vi "PH_Synchrolock_Watch.show Result.vi"(0 "i ref in":refnum<vi>, 1 "RF Current Value":dbl, 2 "Mira Current Value":dbl, 3 "Mean Phase Current Value":dbl, 5 "error in":errorcluster) -> (14 "i ref out":refnum<vi>, 19 "error out":errorcluster)   [LabVIEW 2014, in "PH_Synchrolock_Watch.lvlib"]
doc: "This VI shows the result and stores it at own attributes."
uses:
  PH_Synchrolock_Watch.lvlib
  PH_Basics/PH_Common/PH_Common.lvlib
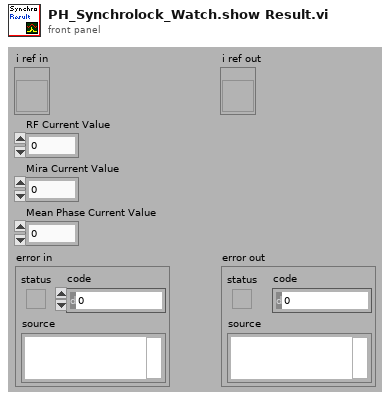
[diagram p1: front panel]
types:
  T1 = typedef "PH_Synchrolock_Watch.lvlib/PH_Synchrolock_Watch.i attribute.ctl" = cluster{"GUI Refs":cluster{"Mean Phase Graph":refnum<vi>, "RF Amplitude Graph":refnum<vi>, "Mira Amplitude Graph":refnum<vi>, "MIRA State":refnum<vi>, "Mean Phase":refnum<vi>, "RF Amplitude":refnum<vi>, "Mira Amplitude":refnum<vi>, "Mean Phase in range?":refnum<vi>, "RF Amplitude above limit?":refnum<vi>, "Mira Amplitude in range?":refnum<vi>, "Mean phase upper limit":refnum<vi>, "Mean phase lower limit":refnum<vi>, "RF Amplitude lower limit":refnum<vi>, "Mira Amplitude lower limit":refnum<vi>, "Mira Amplitude upper limit":refnum<vi>, "Mira scope":refnum<vi>, "Reset Mira warning":refnum<vi>}, "Status":cluster{"Reset Warning":bool}, "Mean Phase":cluster{"Current Value":dbl, "Upper Limit":dbl, "Lower Limit":dbl, "Data":cluster{dbl[], dbl[]}}, "RF":cluster{"Current Value":dbl, "Lower Limit":dbl, "Data":cluster{dbl[], dbl[]}}, "MIRA":cluster{"Current Value":dbl, "Upper Limit":dbl, "Lower Limit":dbl, "Data":cluster{dbl[], dbl[]}}}
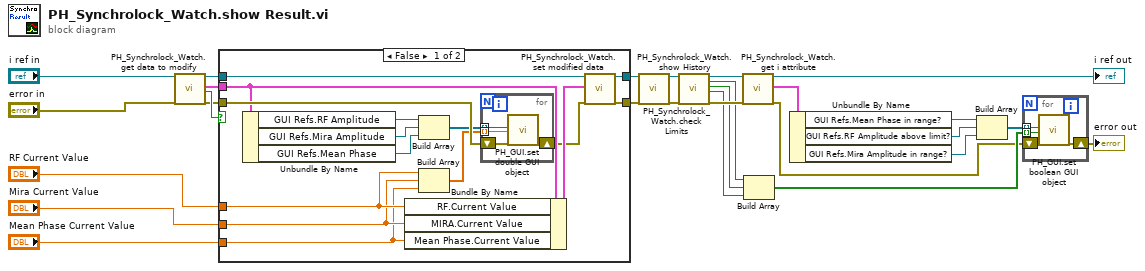
[diagram p0: block diagram]
diagram:
  n1 = call "PH_Synchrolock_Watch.get data to modify.vi"("i ref in"="i ref in", "error in (no error)"="error in") -> ("i ref out"=w23:refnum<vi>, "i attribute"=w27:T1, "timed out"=w26:bool, "error out"=w24:errorcluster)  [unwired: 14 in]
  n2 = case shown="False" w26 {
    tunnel: w23 -> [w42 w48]
    tunnel: [w41 w48] -> w3
    tunnel: w24 -> [w40 w47]
    tunnel: [w39 w47] -> w1
    tunnel: w27 -> [w37 _]
    tunnel: "RF Current Value" -> [w31 _]
    tunnel: "Mira Current Value" -> [w30 _]
    tunnel: "Mean Phase Current Value" -> [w29 _]
    frame False {
      n3 = Unbundle By Name(w37) -> ("GUI Refs.RF Amplitude"=w36:refnum<vi>, "GUI Refs.Mira Amplitude"=w35:refnum<vi>, "GUI Refs.Mean Phase"=w34:refnum<vi>)
      n4 = Bundle By Name(cluster=w37, "RF.Current Value"=w31, "MIRA.Current Value"=w30, "Mean Phase.Current Value"=w29) -> (w38:T1)
      n5 = Build Array(w36, w35, w34) -> (w33:refnum<vi>[])
      n6 = Build Array(w31, w30, w29) -> (w28:dbl[])
      n7 = for {
        shift-right: [w43] -> w32
        shift-left: w40 -> [w46]
        tunnel: w33 -> [w45] mode=indexing
        tunnel: w28 -> [w44] mode=indexing
        n8 = call "PH_GUI.set double GUI object.vi"("GUI object Ref"=w45, "value"=w44, "error in (no error)"=w46) -> ("error out"=w43:errorcluster)  [unwired: 16 in]
      }
      n9 = call "PH_Synchrolock_Watch.set modified data.vi"("i ref in"=w42, "i attribute"=w38, "error in (no error)"=w32) -> ("i ref out"=w41:refnum<vi>, "error out"=w39:errorcluster)  [unwired: 15 in]
    }
    frame True {
    }
  }
  n10 = call "PH_Synchrolock_Watch.show History.vi"("i ref in"=w3, "error in"=w1) -> ("i ref out"=w4:refnum<vi>, "error out"=w2:errorcluster)  [unwired: 16 in]
  n11 = call "PH_Synchrolock_Watch.check Limits.vi"("i ref in"=w4, "error in"=w2) -> ("i ref out"=w16:refnum<vi>, "Phase in range?"=w10:bool, "RF Amplitude below Limit?"=w9:bool, "MIRA Amplitude in range?"=w8:bool, "error out"=w17:errorcluster)  [unwired: 11 in, 2 out]
  n12 = call "PH_Synchrolock_Watch.get i attribute.vi"("i ref in"=w16, "error in (no error)"=w17) -> ("i ref out"=→"i ref out":refnum<vi>, "i attribute"=w11:T1, "error out"=w5:errorcluster)  [unwired: 15 in]
  n13 = Build Array(w10, w9, w8) -> (w6:bool[])
  n14 = Unbundle By Name(w11) -> ("GUI Refs.Mean Phase in range?"=w15:refnum<vi>, "GUI Refs.RF Amplitude above limit?"=w14:refnum<vi>, "GUI Refs.Mira Amplitude in range?"=w13:refnum<vi>)
  n15 = Build Array(w15, w14, w13) -> (w12:refnum<vi>[])
  n16 = for {
    shift-right: [w52] -> w7
    shift-left: w5 -> [w50]
    tunnel: w12 -> [w51] mode=indexing
    tunnel: w6 -> [w49] mode=indexing
    n17 = call "PH_GUI.set boolean GUI object.vi"("Boolean Knob GUI Ref"=w51, "Value"=w49, "error in (no error)"=w50) -> ("error out"=w52:errorcluster)  [unwired: 16 in]
  }
  "error out" <- w7
